vi "ConvertGoop3ToGoop4_ClearErrors.vi"(8 "error in (no error)":errorcluster) -> (0 "error out":errorcluster, 3 "Errors":string[](array[string]))   [LabVIEW 2020]
uses:
  ConvertGoop3ToGoop4_LogType.ctl
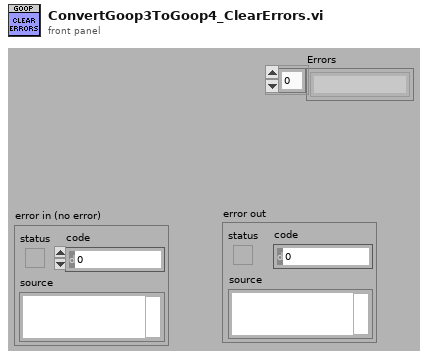
[diagram p1: front panel]
types:
  T1 = typedef "ConvertGoop3ToGoop4_LogType.ctl" = enum16{"Enter", "Read"}
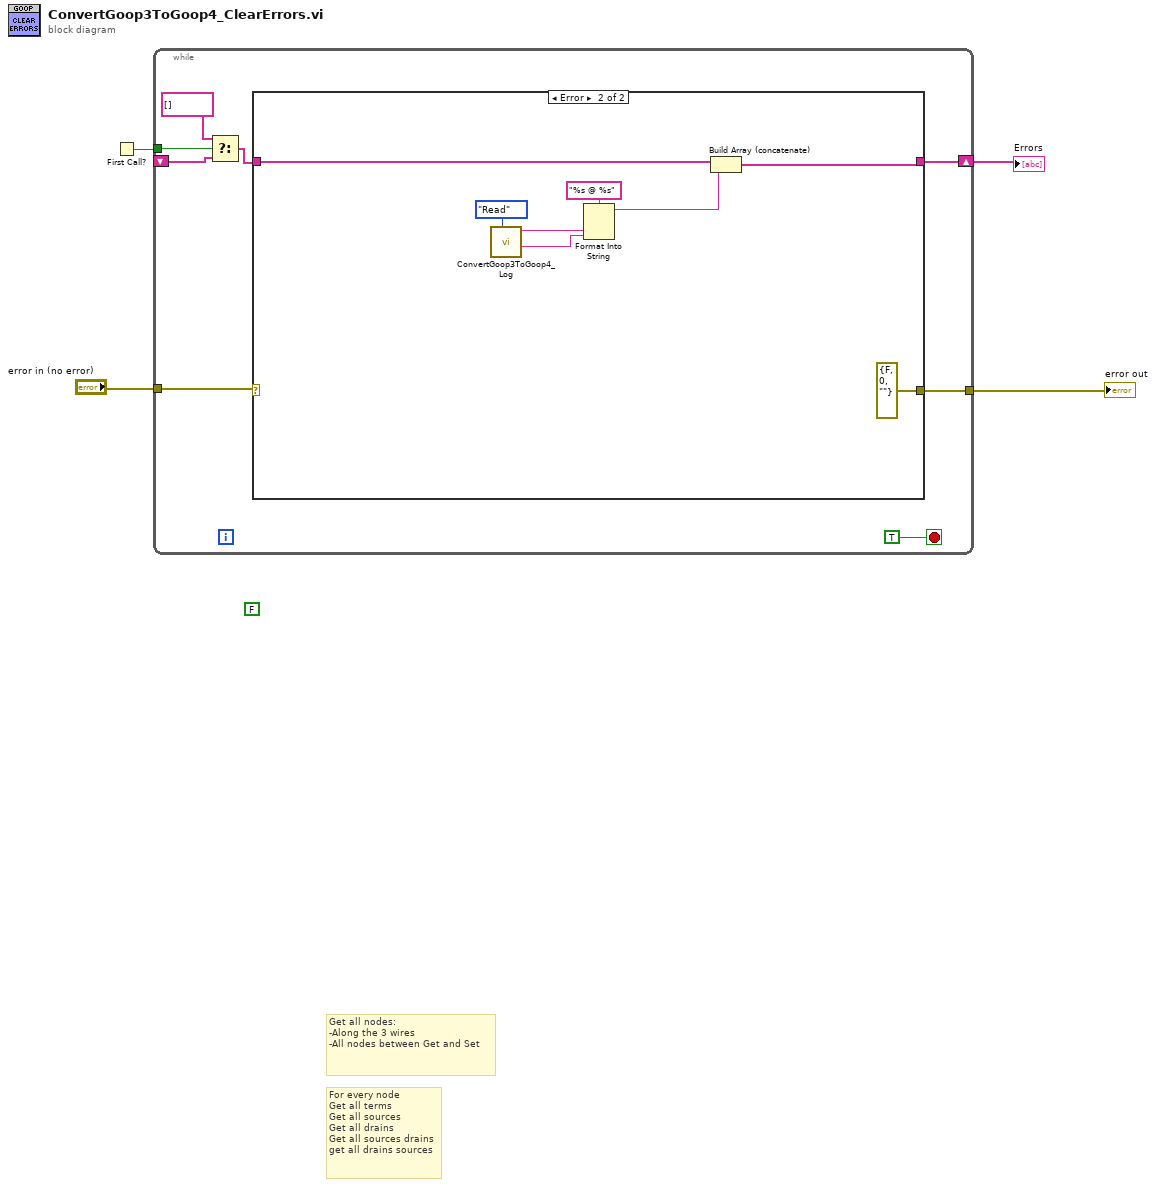
[diagram p0: block diagram]
diagram:
  (unwired) FALSE ("Block Diagram Window:Open")
  # "For every node\nGet all terms\nGet all sources\nGet all drains\nGet all sources drains\nget all drains sources"
  # "Get all nodes:\n-Along the 3 wires\n-All nodes between Get and Set"
  n1 = First Call?() -> (First Call?: T/F=w1:bool)
  n2 = while {
    tunnel: "error in (no error)" -> [w9]
    tunnel: [w12] -> w3
    shift-right: [w10] -> w2
    shift-left: _ -> [w7]
    tunnel: w1 -> [w8]
    stop <- TRUE stop-if-true
    n3 = Select(t=string[] [], s=w8, f=w7) -> (s? t:f=w6:string[])
    n4 = case shown="Error" w9 {
      selector: w9 -> [w14 _]
      tunnel: [w14 errorcluster {"status"=FALSE, "code"=0, "source"=""} ("error IO")] -> w12
      tunnel: [w13 w21] -> w10
      tunnel: w6 -> [w13 w22]
      frame No Error {
      }
      frame Error {
        n5 = call "ConvertGoop3ToGoop4_Log.vi"("Action(Enter)"=ConvertGoop3ToGoop4_LogType."Read") -> ("State"=w18:string, "LastItem"=w19:string)  [unwired: 8 in, 1 out]
        n6 = Format Into String(format string="%s @ %s", w19, w18) -> (resulting string=w16:string)  [unwired: 2 in, 1 out]
        n7 = Build Array (concatenate)(w22, w16) -> (w21:string[])
      }
    }
  }
  "error out" <- w3
  "Errors" <- w2
